vi "raster_array.vi"(8 "x 2":i32, 9 "array":dbl[](array[numeric]), 11 "x":i32) -> (2 "Numeric":dbl)   [LabVIEW 2014]
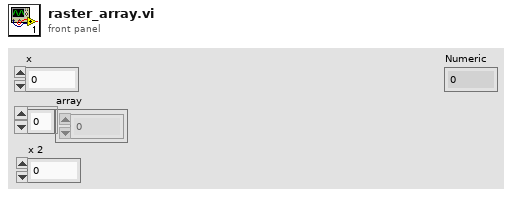
[diagram p1: front panel]
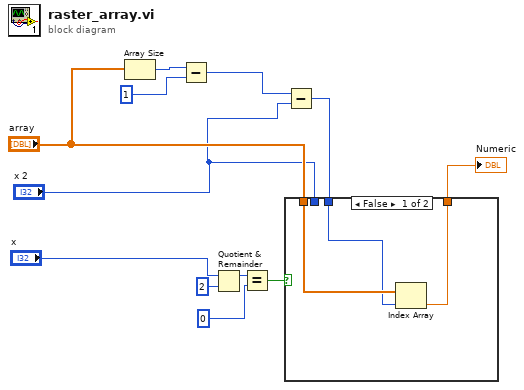
[diagram p0: block diagram]
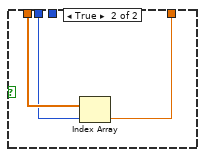
[diagram p2: hidden frame]
diagram:
  n1 = Array Size(array="array") -> (size(s)=w7:i32)
  n2 = Subtract(x=w7, y=1) -> (x-y=w6:i32)
  n3 = Quotient & Remainder(x="x", y=2) -> (x-y*floor(x/y)=w11:i32)  [unwired: 1 out]
  n4 = Equal?(x=w11, y=0) -> (x = y?=w9:bool)
  n5 = Subtract(x=w6, y="x 2") -> (x-y=w5:i32)
  n6 = case shown="False" w9 {
    tunnel: "array" -> [w14 w18]
    tunnel: "x 2" -> [_ w17]
    tunnel: [w15 w16] -> w2
    tunnel: w5 -> [w13 _]
    frame False {
      n7 = Index Array(array=w14, index=w13) -> (element=w15:dbl)
    }
    frame True {
      n8 = Index Array(array=w18, index=w17) -> (element=w16:dbl)
    }
  }
  "Numeric" <- w2
